vi "Autosize Listbox Columns (Uniform Text).vi"(4 "error in (no error)":errorcluster, 5 "y 2":dbl=1.2, 6 "Resize Table?":bool, 7 "reference In":refnum<vi>) -> (0 "error out":errorcluster, 3 "reference Out":refnum<vi>)   [LabVIEW 2021]
doc: "This VI resizes each column of the table specified by Table Ref based on the widest entry of the column. Additionally, if Resize Table? is TRUE, the VI will set the table width based on the number of populated columns."
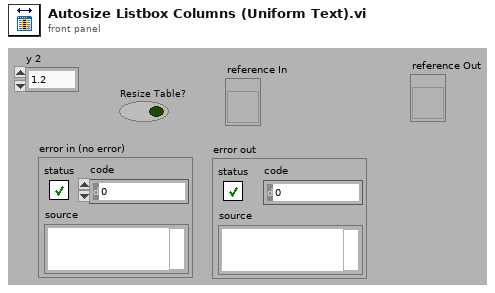
[diagram p1: front panel]
types:
  T1 = enum16{"User-specified Font", "Application Font", "System Font", "Dialog Font"}
  T2 = cluster{"Font Name:":string, "Size":i16, "Strikeout?":bool, "Italic?":bool, "Underline?":bool, "Outline?":bool, "Shadow?":bool, "Bold?":bool}
  T3 = cluster{"left":i16, "top":i16, "right":i16, "bottom":i16}
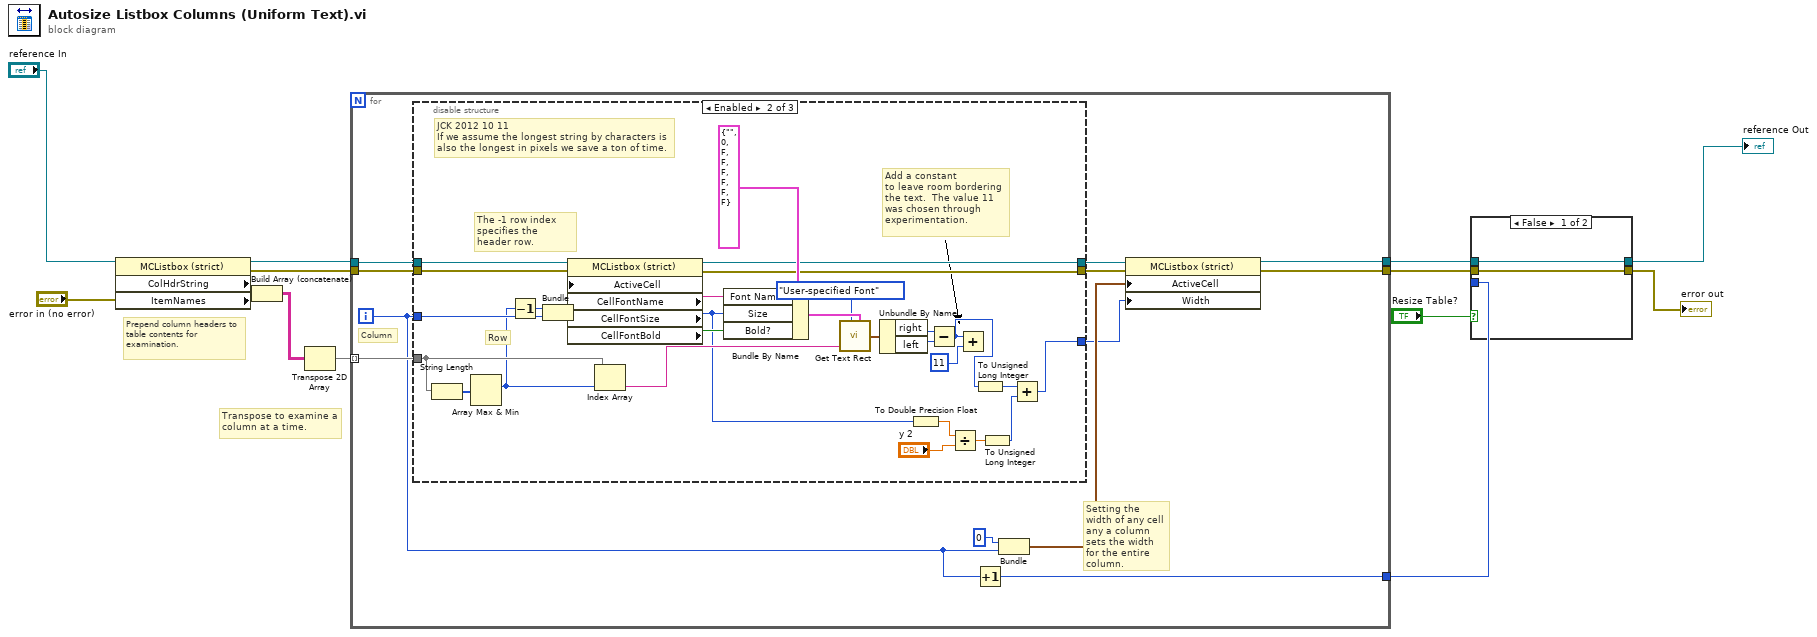
[diagram p0: block diagram]
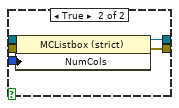
[diagram p2: hidden frame]
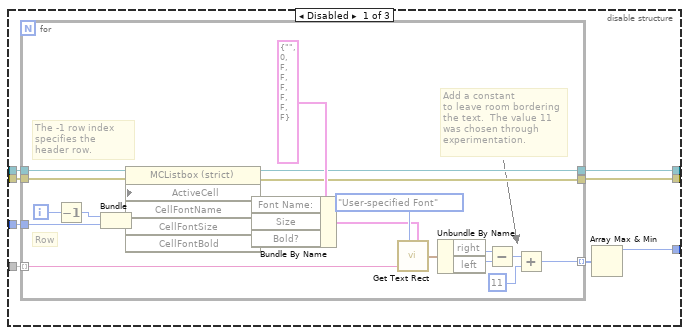
[diagram p3: hidden frame]
diagram:
  # "Transpose to examine a column at a time."
  # "Prepend column headers to table contents for examination."
  n1 = property class="MCListbox (strict)"(reference="reference In", error in="error in (no error)") -> (reference out=w14:refnum<vi>, error out=w10:errorcluster, "ColHdrString"=w13:string[], "ItemNames"=w9:string[][])
  n2 = Build Array (concatenate)(w13, w9) -> (w12:string[][])
  n3 = Transpose 2D Array(2D array=w12) -> (transposed array=w11:string[][])
  n4 = for {
    tunnel: w11 -> [w26] mode=indexing
    tunnel: w14 -> [w25]
    tunnel: w10 -> [w24]
    tunnel: [w18] -> w5
    tunnel: [w17] -> w6
    tunnel: [w15] -> w4
    i -> [w16]
    # "Setting the width of any cell any a column sets the width for the entire column."
    # "Column"
    n5 = disable-structure shown="Enabled" {
      disable-tunnel: w26 -> [w34 w70 _]
      disable-tunnel: w25 -> [w33 w67 _]
      disable-tunnel: w24 -> [w31 w66 _]
      disable-tunnel: [w30 w65 _] -> w23
      disable-tunnel: [w29 w64 _] -> w22
      disable-tunnel: [w28 w56 _] -> w19
      disable-tunnel: w16 -> [w27 w71 _]
      frame Disabled {
        n6 = for {
          tunnel: w34 -> [w47] mode=indexing
          tunnel: w33 -> [w55]
          tunnel: w27 -> [w54]
          tunnel: [w36] -> w32 mode=indexing
          tunnel: w31 -> [w41]
          tunnel: [w40] -> w29
          tunnel: [w39] -> w30
          i -> [w43]
          # "The -1 row index specifies the header row."
          # "Add a constant\nto leave room bordering the text.  The value 11 was chosen through experimentation."
          # "Row"
          n7 = Decrement(x=w43) -> (x-1=w42:i32)
          n8 = Bundle(w42, w54) -> (w53:cluster{i32, i32})  [unwired: 1 in]
          n9 = property class="MCListbox (strict)"(reference=w55, error in=w41, "ActiveCell"=w53) -> (reference out=w39:refnum<vi>, error out=w40:errorcluster, "CellFontName"=w51:string, "CellFontSize"=w37:u32, "CellFontBold"=w50:bool)
          n10 = Bundle By Name(cluster=T2 {"Font Name:"="", "Size"=0, "Strikeout?"=FALSE, "Italic?"=FALSE, "Underline?"=FALSE, "Outline?"=FALSE, "Shadow?"=FALSE, "Bold?"=FALSE} ("[user-specified font]"), "Font Name:"=w51, "Size"=w37, "Bold?"=w50) -> (w48:T2)
          n11 = call <vilib>:"Get Text Rect.vi"("desired font(Application)"=T1."User-specified Font", "text"=w47, "[user-specified font]"=w48) -> ("rect"=w46:T3)  [unwired: 6 in]
          n12 = Unbundle By Name(w46) -> ("right"=w45:i16, "left"=w44:i16)
          n13 = Subtract(x=w45, y=w44) -> (x-y=w38:i16)
          n14 = Add(x=w38, y=i16 11) -> (x+y=w36:i16)
        }
        n15 = Array Max & Min(array=w32) -> (max value=w28:i16)  [unwired: 3 out]
      }
      frame Enabled {
        # "JCK 2012 10 11\nIf we assume the longest string by characters is also the longest in pixels we save a ton of time."
        # "The -1 row index specifies the header row."
        # "Add a constant\nto leave room bordering the text.  The value 11 was chosen through experimentation."
        # "Row"
        n16 = String Length(string=w70) -> (length=w83:i32[])
        n17 = Array Max & Min(array=w83) -> (max index (indices)=w69:i32)  [unwired: 3 out]
        n18 = Decrement(x=w69) -> (x-1=w81:i32)
        n19 = Bundle(w81, w71) -> (w72:cluster{i32, i32})  [unwired: 1 in]
        n20 = property class="MCListbox (strict)"(reference=w67, error in=w66, "ActiveCell"=w72) -> (reference out=w65:refnum<vi>, error out=w64:errorcluster, "CellFontName"=w74:string, "CellFontSize"=w57:u32, "CellFontBold"=w75:bool)
        n21 = Index Array(array=w70, index=w69) -> (element=w68:string)
        n22 = Bundle By Name(cluster=T2 {"Font Name:"="", "Size"=0, "Strikeout?"=FALSE, "Italic?"=FALSE, "Underline?"=FALSE, "Outline?"=FALSE, "Shadow?"=FALSE, "Bold?"=FALSE} ("[user-specified font]"), "Font Name:"=w74, "Size"=w57, "Bold?"=w75) -> (w77:T2)
        n23 = call <vilib>:"Get Text Rect.vi"("desired font(Application)"=T1."User-specified Font", "text"=w68, "[user-specified font]"=w77) -> ("rect"=w78:T3)  [unwired: 6 in]
        n24 = Unbundle By Name(w78) -> ("right"=w79:i16, "left"=w80:i16)
        n25 = To Double Precision Float(number=w57) -> (double precision float=w59:dbl)
        n26 = Subtract(x=w79, y=w80) -> (x-y=w58:i16)
        n27 = Divide(x=w59, y="y 2") -> (x/y=w61:dbl)
        n28 = Add(x=w58, y=i16 11) -> ()  [unwired: 1 out]
        n29 = To Unsigned Long Integer(number=w58) -> (unsigned 32bit integer=w62:u32)
        n30 = To Unsigned Long Integer(number=w61) -> (unsigned 32bit integer=w63:u32)
        n31 = Add(x=w62, y=w63) -> (x+y=w56:u32)
      }
      frame Disabled {
      }
    }
    n32 = Increment(x=w16) -> (x+1=w15:i32)
    n33 = Bundle(0, w16) -> (w20:cluster{i32, i32})  [unwired: 1 in]
    n34 = property class="MCListbox (strict)"(reference=w23, error in=w22, "ActiveCell"=w20, "Width"=w19) -> (reference out=w17:refnum<vi>, error out=w18:errorcluster)
  }
  n35 = case shown="False" "Resize Table?" {
    tunnel: w6 -> [w84 w90]
    tunnel: w5 -> [w85 w89]
    tunnel: w4 -> [_ w88]
    tunnel: [w85 w87] -> w3
    tunnel: [w84 w86] -> w1
    frame False {
    }
    frame True {
      n36 = property class="MCListbox (strict)"(reference=w90, error in=w89, "NumCols"=w88) -> (reference out=w86:refnum<vi>, error out=w87:errorcluster)
    }
  }
  "error out" <- w3
  "reference Out" <- w1
